vi "Digital Compass.vi"() -> ()   [LabVIEW 2012]
uses:
  <vilib>/Math Plots/2D Math Plots/2D Compass/2D Compass XCtrl/2D Compass.xctl
  <vilib>/LabVIEW Interface for Arduino/Type Defs/Connection Type.ctl
  <vilib>/LabVIEW Interface for Arduino/Type Defs/Board Type.ctl
  <vilib>/Math Plots/2D Math Plots/2D Compass/2D Compass Datatype/Public/Plot Helper (Vector).vi
  <vilib>/Math Plots/2D Math Plots/2D Compass/2D Compass Datatype/2D Compass Datatype.lvclass
  <vilib>/LabVIEW Interface for Arduino/LabVIEW Interface for Arduino.lvlib
panel:
  out "output array":dbl[](array[numeric])
  out "I2C Data":u8[](array[numeric])
  in  "stop":bool
  out "2D Compass":refnum<class "2D Plot Datatype.lvclass">[](xcontrol)
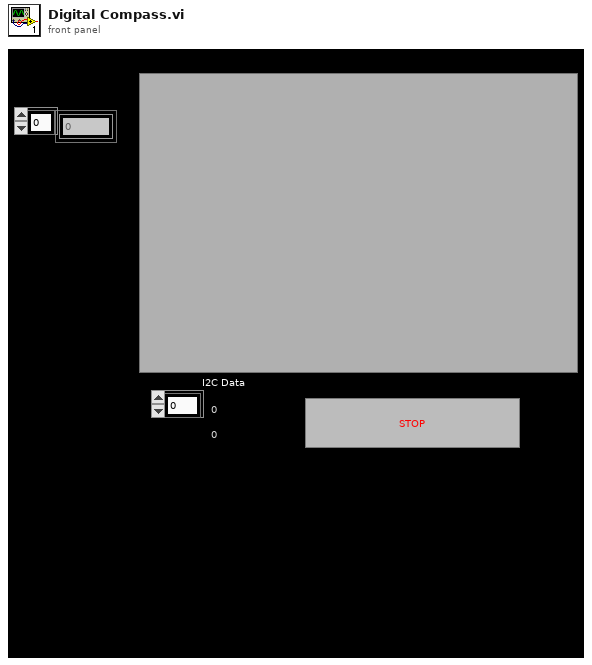
[diagram p1: front panel]
types:
  T1 = typedef "LabVIEW Interface for Arduino.lvlib/Board Type.ctl" = enum16{"Uno", "Dimuelanove w/Atmega 328", "Mega 2560"}
  T2 = typedef "LabVIEW Interface for Arduino.lvlib/Connection Type.ctl" = enum8{"USB / Serial", "XBEE", "BlueSmirf (Bluetooth)"}
  T3 = typedef "LabVIEW Interface for Arduino.lvlib/Arduino Resource.ctl" = cluster{"VISA resource":refnum<visa-resource-name>, "Board Type":T1, "Connection Type":enum8{"USB / Serial"}, "Bytes Per Packet (15)":u8}
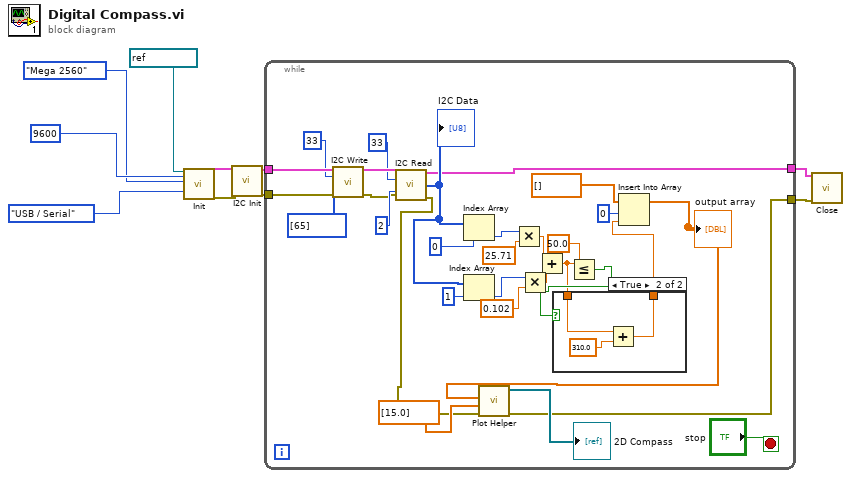
[diagram p0: block diagram]
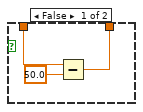
[diagram p2: hidden frame]
diagram:
  n1 = call <vilib>:"Init.vi"("VISA resource"=refnum<visa-resource-name> "COM11", "Baud Rate (115200)"=u32 9600, "Board Type (Uno)"=Board_Type."Mega 2560", "Connection Type (USB/Serial)"=Connection_Type."USB / Serial") -> ("Arduino Resource"=w10:T3, "error out"=w9:errorcluster)  [unwired: 14 in]
  n2 = call <vilib>:"I2C Init.vi"("Arduino Resource"=w10, "error in"=w9) -> ("Arduino Resource"=w8:T3, "error out"=w7:errorcluster)  [unwired: 12 in]
  n3 = while {
    tunnel: w8 -> [w39]
    tunnel: w7 -> [w38]
    tunnel: [w23] -> w6
    tunnel: [w22] -> w5
    stop <- "stop" stop-if-true
    n4 = call <vilib>:"I2C Write.vi"("Arduino Resource"=w39, "Address (0)"=u8 33, "I2C Data Bytes"=u8[] [65], "error in"=w38) -> ("Arduino Resource"=w33:T3, "error out"=w34:errorcluster)  [unwired: 10 in]
    n5 = call <vilib>:"I2C Read.vi"("Arduino Resource"=w33, "Address (0)"=u8 33, "Bytes To Read"=u8 2, "error in"=w34) -> ("Arduino Resource"=w23:T3, "I2C Data"=w29:u8[], "error out"=w24:errorcluster)  [unwired: 9 in]
    "I2C Data" <- w29
    n6 = Index Array(array=w29, index=0) -> (element=w21:u8)
    n7 = Index Array(array=w29, index=1) -> (element=w19:u8)
    n8 = Multiply(x=w21, y=25.71) -> (x*y=w17:dbl)
    n9 = Multiply(x=w19, y=0.102) -> (x*y=w16:dbl)
    n10 = Add(x=w17, y=w16) -> (x+y=w12:dbl)
    n11 = Less Or Equal?(x=w12, y=50.0) -> (x <= y?=w13:bool)
    n12 = case shown="True" w13 {
      tunnel: w12 -> [w43 w46]
      tunnel: [w41 w45] -> w11
      frame False {
        n13 = Subtract(x=w43, y=50.0) -> (x-y=w41:dbl)
      }
      frame True {
        n14 = Add(x=w46, y=310.0) -> (x+y=w45:dbl)
      }
    }
    n15 = Insert Into Array(array=dbl[] [], index=0, new element=w11) -> (w15:dbl[])
    "output array" <- w15
    n16 = call-poly <vilib>:"Plot Helper.vi"("error in (no error)"=w24, "radius vector"=dbl[] [15.0], "theta vector"=w15) -> ("error out"=w22:errorcluster, "2D Plot Class Obj Array out"=→"2D Compass":refnum<class "2D Plot Datatype.lvclass">[])  [unwired: 1 in, 6 out]
  }
  n17 = call <vilib>:"Close.vi"("Arduino Resource"=w6, "error in"=w5) -> ()  [unwired: 13 in, 1 out]
